vi "WriteRegs.vi"(0 "VISA Refnum in":refnum<visa-resource-name>, 1 "StartAddr":u16, 3 "DataArray":u16[](array[numeric]), 5 "Cluster":T1, 11 "error in":errorcluster) -> (4 "VISA out":refnum<visa-resource-name>, 6 "Cluster Out":T1, 15 "error out":errorcluster)   [LabVIEW 2020]
uses:
  <vilib>/NI Modbus.llb/MB Serial Master Query Write Multiple Registers (poly).vi
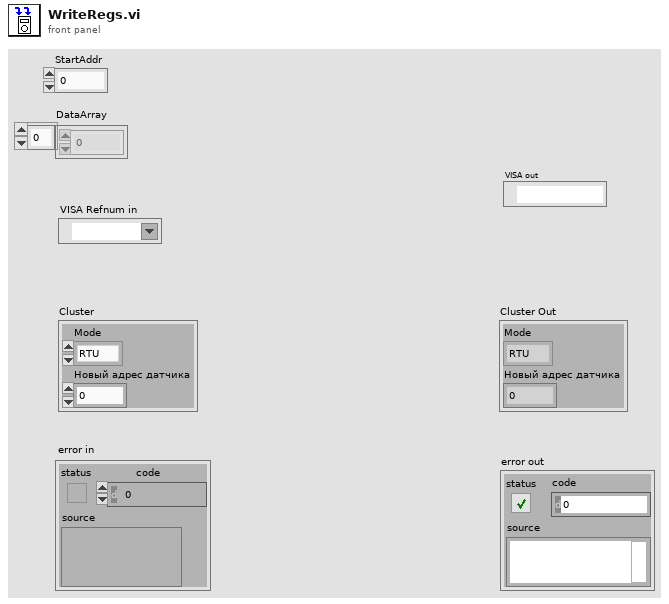
[diagram p1: front panel]
types:
  T1 = cluster{"Mode":enum16{"RTU", "ASCII"}, "Новый адрес датчика":u16}
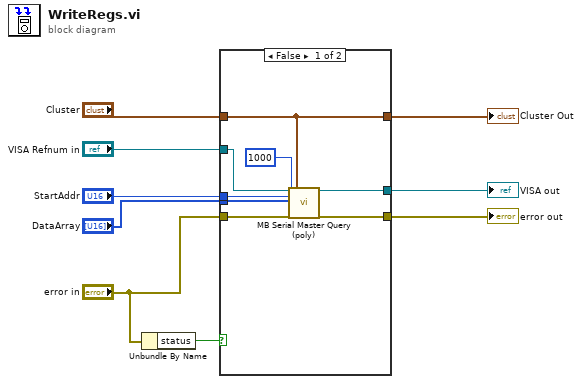
[diagram p0: block diagram]
diagram:
  n1 = Unbundle By Name("error in") -> ("status"=w3:bool)
  n2 = case shown="False" w3 {
    tunnel: "VISA Refnum in" -> [w17 w18]
    tunnel: "DataArray" -> [w16 _]
    tunnel: "error in" -> [w15 w20]
    tunnel: "StartAddr" -> [w14 _]
    tunnel: [w13 w18] -> w7
    tunnel: [w12 w20] -> w6
    tunnel: "Cluster" -> [w11 w19]
    tunnel: [w11 w19] -> w2
    frame False {
      n3 = call-poly <vilib>:"MB Serial Master Query (poly).vi"("VISA resource name"=w17, "Starting Address"=w14, "Registers"=w16, "Timeout"=u32 1000, "error in"=w15, "Serial Parameters"=w11) -> ("VISA resource name out"=w13:refnum<visa-resource-name>, "error out"=w12:errorcluster)  [unwired: 12 out]
    }
    frame True {
    }
  }
  "error out" <- w6
  "VISA out" <- w7
  "Cluster Out" <- w2
